vi "Parse Message.vi"(8 "error in (no error)":errorcluster, 10 "Data":string, 11 "OBS in":refnum<class "OBS.lvclass">) -> (0 "error out":errorcluster, 2 "Server Message":refnum<class "Server Message.lvclass">, 3 "OBS out":refnum<class "OBS.lvclass">)   [LabVIEW 2022 SP3, in "obs-websocket-lv.lvlib" / "OBS.lvclass"]
uses:
  OBS.lvclass
  Server Message/Server Message.lvclass
  Hello/Hello.lvclass
  C:/dev/illuminatedg/obs-websocket-lv/obs-websocket-lv/Server Message/Server Message.lvclass
  Identified/Identified.lvclass
  Event/Event.lvclass
  Response/Response.lvclass
  BatchResponse/BatchResponse.lvclass
  OBS.lvclass/OBS.ctl
  <vilib>/IlluminatedG/lv-web-crypto/lv-json/JSON/JSON.lvlib
  obs-websocket-lv.lvlib
  C:/dev/illuminatedg/obs-websocket-lv/obs-websocket-lv/Message/Message.lvclass
  C:/dev/illuminatedg/obs-websocket-lv/obs-websocket-lv/Response/Response.lvclass
  C:/dev/illuminatedg/obs-websocket-lv/obs-websocket-lv/Hello/Hello.lvclass
  C:/dev/illuminatedg/obs-websocket-lv/obs-websocket-lv/Identified/Identified.lvclass
  C:/dev/illuminatedg/obs-websocket-lv/obs-websocket-lv/Event/Event.lvclass
  C:/dev/illuminatedg/obs-websocket-lv/obs-websocket-lv/BatchResponse/BatchResponse.lvclass
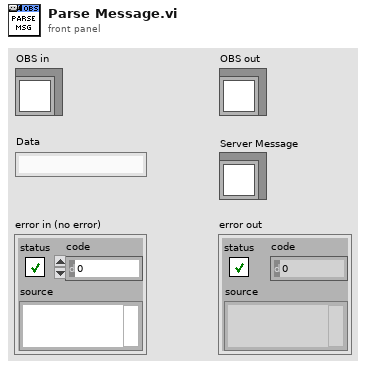
[diagram p1: front panel]
types:
  T1 = typedef "JSON.lvlib/JSON Item Type.ctl" = enum16{"unknown", "null", "Array", "Object", "String", "Number", "Boolean"}
  T2 = typedef "obs-websocket-lv.lvlib/Server Operation.ctl" = enum16{"Hello", "Identified", "Event", "RequestResponse", "RequestBatchResponse"}
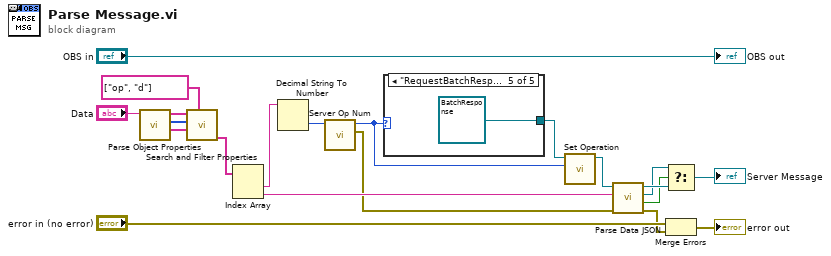
[diagram p0: block diagram]
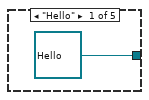
[diagram p2: hidden frame]
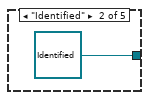
[diagram p3: hidden frame]
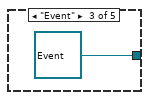
[diagram p4: hidden frame]
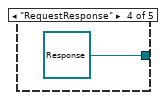
[diagram p5: hidden frame]
diagram:
  n1 = call <vilib>:"Parse Object Properties.vi"("JSON String"="Data") -> ("Values"=w16:string[], "Item Types"=w17:T1[], "Keys"=w18:string[])  [unwired: 7 in, 1 out]
  n2 = call <vilib>:"Search and Filter Properties.vi"("Search Keys"=string[] ["op", "d"], "Values In"=w16, "Types In"=w17, "Keys In"=w18) -> ("Filtered Values"=w14:string[])  [unwired: 2 in, 5 out]
  n3 = Index Array(array=w14) -> (element #1=w13:string, element #2=w12:string)  [unwired: 2 in]
  n4 = Decimal String To Number(string=w13) -> (number=w9:i32)  [unwired: 2 in, 1 out]
  n5 = call "Server Op Num.vi"("Server Op Num"=w9) -> ("error out"=w8:errorcluster, "Server Operation"=w5:T2)  [unwired: 9 in]
  n6 = case shown="\"RequestBatchResponse\"" w5 {
    tunnel: [refnum<class "Hello.lvclass"> refnum ("obs-websocket-lv.lvlib:Hello.lvclass") refnum<class "Identified.lvclass"> refnum ("obs-websocket-lv.lvlib:Identified.lvclass") refnum<class "Event.lvclass"> refnum ("obs-websocket-lv.lvlib:Event.lvclass") refnum<class "Response.lvclass"> refnum ("obs-websocket-lv.lvlib:Response.lvclass") refnum<class "BatchResponse.lvclass"> refnum ("obs-websocket-lv.lvlib:BatchResponse.lvclass")] -> w6
    frame "Hello" {
    }
    frame "Identified" {
    }
    frame "Event" {
    }
    frame "RequestResponse" {
    }
    frame "RequestBatchResponse" {
    }
  }
  n7 = call "Set Operation.vi"("Server Operation"=w5, "Server Message in"=w6) -> ("Server Message out"=w7:refnum<class "Server Message.lvclass">)  [unwired: 8 in, 1 out]
  n8 = call-dynamic "Parse Data JSON.vi"("error in (no error)"=w8, "Data JSON"=w12, "Server Message in"=w7) -> ("error out"=w10:errorcluster, "Replaced?"=w2:bool, "Typed Message"=w3:refnum<class "Response.lvclass">, "Server Message out"=w4:refnum<class "Server Message.lvclass">)  [unwired: 5 in]
  n9 = Select(t=w3, s=w2, f=w4) -> (s? t:f=→"Server Message":refnum<class "Server Message.lvclass">)
  n10 = Merge Errors("error in (no error)", w10) -> (→"error out":errorcluster)
  "OBS out" <- "OBS in"
